vi "svl_Check Calibration Parameters.vi"(0 "frequency tolerance [%]":dbl format="%.2f", 5 "sampling frequency [Hz]":dbl format="%.2f", 7 "duration [s]":dbl format="%.2f", 9 "calibration frequency [Hz]":dbl format="%.2f", 11 "error in (no error)":errorcluster) -> (4 "dup frequency tolerance [%]":dbl format="%.2f", 6 "dup sampling frequency [Hz]":dbl format="%.2f", 8 "dup duration [s]":dbl format="%.2f", 10 "dup calibration frequency [Hz]":dbl format="%.2f", 15 "error out":errorcluster)   [LabVIEW 2017, in "SoundVib_Calibration.lvlib"]
uses:
  <vilib>/addons/Sound and Vibration/svt_Calibration/SoundVib_Calibration.lvlib
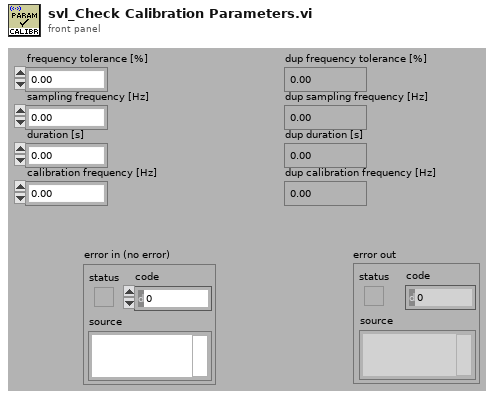
[diagram p1: front panel]
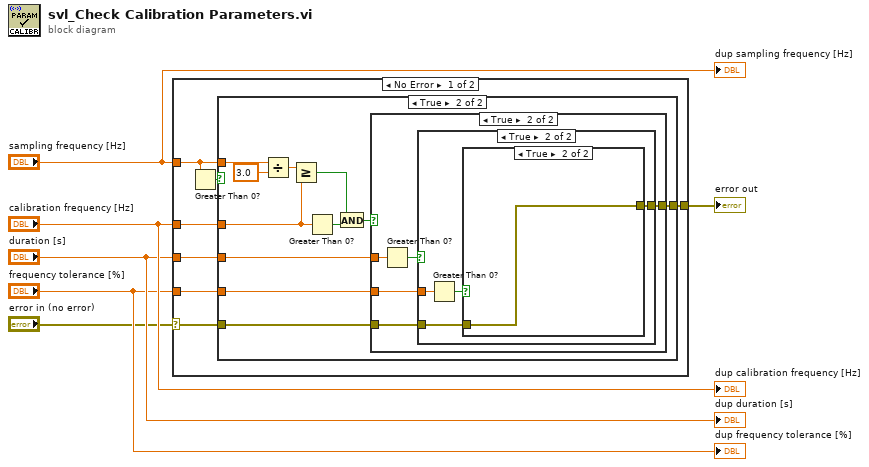
[diagram p0: block diagram]
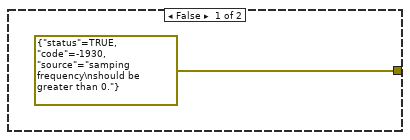
[diagram p2: hidden frame]
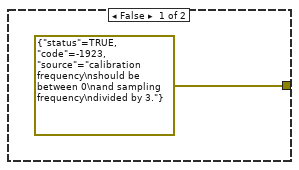
[diagram p3: hidden frame]
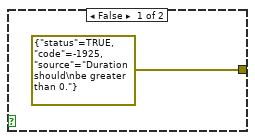
[diagram p4: hidden frame]
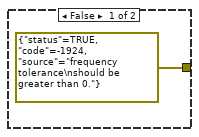
[diagram p5: hidden frame]
diagram:
  n1 = case shown="No Error" "error in (no error)" {
    selector: "error in (no error)" -> [w7 w39]
    tunnel: [w12 w39] -> w6
    tunnel: "sampling frequency [Hz]" -> [w11 _]
    tunnel: "calibration frequency [Hz]" -> [w10 _]
    tunnel: "duration [s]" -> [w9 _]
    tunnel: "frequency tolerance [%]" -> [w8 _]
    frame No Error {
      n2 = Greater Than 0?(x=w11) -> (x > 0?=w13:bool)
      n3 = case shown="True" w13 {
        tunnel: w8 -> [_ w25]
        tunnel: w10 -> [_ w19]
        tunnel: w9 -> [_ w24]
        tunnel: w11 -> [_ w20]
        tunnel: [errorcluster {"status"=TRUE, "code"=-1930, "source"="samping frequency\nshould be greater than 0."} ("error out") w23] -> w12
        tunnel: w7 -> [_ w15]
        frame False {
        }
        frame True {
          n4 = Divide(x=w20, y=3.0) -> (x/y=w22:dbl)
          n5 = Greater Or Equal?(x=w22, y=w19) -> (x >= y?=w16:bool)
          n6 = Greater Than 0?(x=w19) -> (x > 0?=w17:bool)
          n7 = And(x=w16, y=w17) -> (x .and. y?=w18:bool)
          n8 = case shown="True" w18 {
            tunnel: w25 -> [_ w31]
            tunnel: w24 -> [_ w29]
            tunnel: [errorcluster {"status"=TRUE, "code"=-1923, "source"="calibration frequency\nshould be between 0\nand sampling frequency\ndivided by 3."} ("error out") w30] -> w23
            tunnel: w15 -> [_ w27]
            frame False {
            }
            frame True {
              n9 = Greater Than 0?(x=w29) -> (x > 0?=w28:bool)
              n10 = case shown="True" w28 {
                tunnel: w31 -> [_ w36]
                tunnel: [errorcluster {"status"=TRUE, "code"=-1925, "source"="Duration should\nbe greater than 0."} ("error out") w34] -> w30
                tunnel: w27 -> [_ w33]
                frame False {
                }
                frame True {
                  n11 = Greater Than 0?(x=w36) -> (x > 0?=w35:bool)
                  n12 = case shown="True" w35 {
                    tunnel: [errorcluster {"status"=TRUE, "code"=-1924, "source"="frequency tolerance\nshould be greater than 0."} ("error out") w38] -> w34
                    tunnel: w33 -> [_ w38]
                    frame False {
                    }
                    frame True {
                    }
                  }
                }
              }
            }
          }
        }
      }
    }
    frame Error {
    }
  }
  "error out" <- w6
  "dup frequency tolerance [%]" <- "frequency tolerance [%]"
  "dup duration [s]" <- "duration [s]"
  "dup calibration frequency [Hz]" <- "calibration frequency [Hz]"
  "dup sampling frequency [Hz]" <- "sampling frequency [Hz]"
